vi "NewtonsPSM_Conf_Sweep.vi"(0 "VISA session":refnum<visa-resource-name>, 1 "Steps (Log)":u16(ring) items=["Log", "Linear"], 2 "Sweep (Single)":u16(ring) items=["Single", "Repeat"], 5 "error in (no error)":errorcluster, 6 "Steps (32)":u8=32 min=2 max=64 step=1, 7 "Frequency Market (Off)":bool, 9 "Sweep Start (1000)":dbl=1000.0 min=0.0 max=35000000.0 step=1e-05, 11 "Sweep Stop (1000000)":sgl=1000000.0 max=3.5e+07) -> (14 "dup VISA session":refnum<visa-resource-name>, 19 "error out":errorcluster)   [LabVIEW 2025, in "NewtonsPSM1735.lvlib"]
doc: "This VI set the Scope mode parameters to the PPA2530\nTrigger parameters and Time Base"
uses:
  NewtonsPSM1735.lvlib
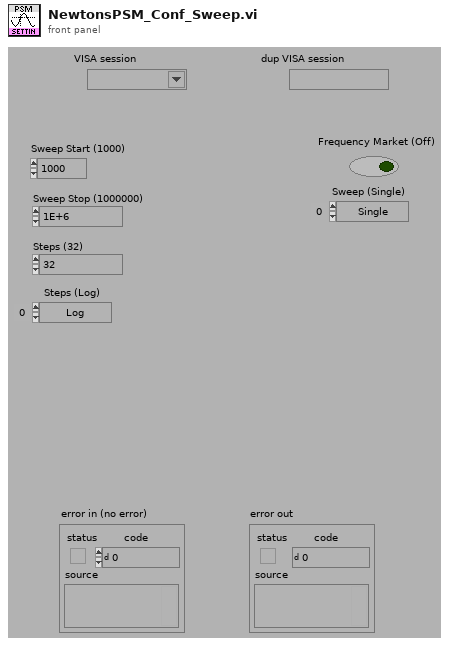
[diagram p1: front panel]
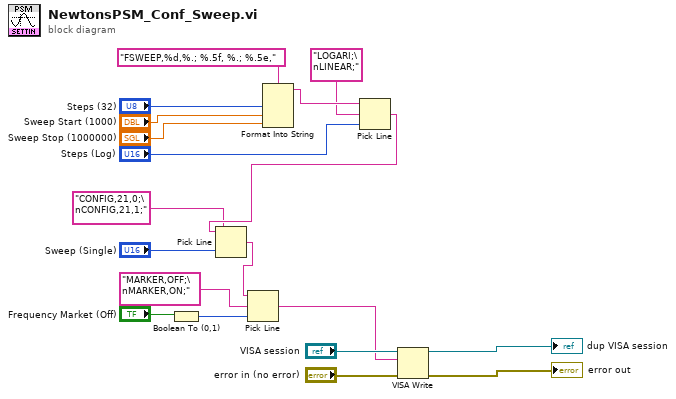
[diagram p0: block diagram]
diagram:
  n1 = Boolean To (0,1)(Boolean="Frequency Market (Off)") -> (0, 1=w4:i16)
  n2 = Format Into String(format string="FSWEEP,%d,%.; %.5f, %.; %.5e,", "Steps (32)", "Sweep Start (1000)", "Sweep Stop (1000000)") -> (resulting string=w11:string)  [unwired: 2 in, 1 out]
  n3 = Pick Line(string ("")=w11, multi-line string="LOGARI;\nLINEAR;", line index="Steps (Log)") -> (output string=w7:string)
  n4 = Pick Line(string ("")=w7, multi-line string="CONFIG,21,0;\nCONFIG,21,1;" ("chaîne multiligne"), line index="Sweep (Single)") -> (output string=w3:string)
  n5 = Pick Line(string ("")=w3, multi-line string="MARKER,OFF;\nMARKER,ON;" ("chaîne multiligne"), line index=w4) -> (output string=w1:string)
  n6 = VISA Write(VISA resource name="VISA session", write buffer=w1, error in (no error)="error in (no error)") -> (VISA resource name out=→"dup VISA session":refnum<visa-resource-name>, error out=→"error out":errorcluster)  [unwired: 1 out]
